vi "Test Drive.vi"   [LabVIEW 2016]
uses:
  <vilib>/Rock Robotics/WPI/ThirdParty/CanMotor/TalonSRX/WPI_CANTalonSRX_APIControlMode.ctl
  <vilib>/Rock Robotics/WPI/Solenoid/WPI_SolenoidValue.ctl
  Global Variables/Refnum Names.vi
  <vilib>/Rock Robotics/WPI/Utilities/WPI_GetSetVariantRefNum.vi
  <vilib>/Rock Robotics/WPI/Joystick/WPI_JoystickArcadeMapping.vi
  <vilib>/Rock Robotics/WPI/Solenoid/WPI_SolenoidSetEnum.vi
types:
  T1 = typedef "WPI_CANTalonSRX_APIControlMode.ctl" = enum8{"Percent VBus", "Speed", "Position", "Slave", "Unchanged / Invalid", "Voltage Compensation", "Current", "Motion Profile", "Motion Magic"}
  T2 = typedef "WPI_MotorControlDeviceRef.ctl" = cluster{"DeviceStatus":errorcluster, "Type":T3, "PWM":cluster{"PWM Channel":T4, "DeadBand":T5}, "CAN":cluster{"Device Number":u8, "SetOutput VI Ref":variant, "GetOutput VI Ref":variant, "Enable VI Ref":variant, "Disable VI Ref":variant, "Data":variant}, "Invert":bool}
  T3 = typedef "WPI_MotorControlType.ctl" = enum16{"PWM", "CAN"}
  T4 = typedef "FPGA_DIOPWMChannel.ctl" = enum8{"PWM 0", "PWM 1", "PWM 2", "PWM 3", "PWM 4", "PWM 5", "PWM 6", "PWM 7", "PWM 8", "PWM 9", "PWM MXP 0", "PWM MXP 1", "PWM MXP 2", "PWM MXP 3", "PWM MXP 4", "PWM MXP 5", "PWM MXP 6", "PWM MXP 7", "PWM MXP 8", "PWM MXP 9", "Invalid"}
  T5 = typedef "WPI_PWMDeadband.ctl" = cluster{"Name":string, "maxPositivePwm":i32, "minPositivePwm":i32, "centerPwm":i32, "maxNegativePwm":i32, "minNegativePwm":i32, "angularRange":u16}
  T6 = typedef "WPI_JoystickDevRef.ctl" = cluster{"Device":T7}
  T7 = typedef "WPI_JoystickDeviceEnum.ctl" = enum16{"USB 0", "USB 1", "USB 2", "USB 3", "USB 4", "USB 5"}
  T8 = typedef "WPI_SolenoidDevRef.ctl" = cluster{"DevStatus":errorcluster, "Pneumatics Control Module":u8, "Forward Solenoid Channel":T9, "Reverse Solenoid Channel":T9}
  T9 = typedef "WPI_SolenoidChannel.ctl" = enum8{"Solenoid 0", "Solenoid 1", "Solenoid 2", "Solenoid 3", "Solenoid 4", "Solenoid 5", "Solenoid 6", "Solenoid 7", "Invalid"}
  T10 = typedef "WPI_SolenoidValue.ctl" = enum16{"Off", "On", "Forward", "Reverse"}
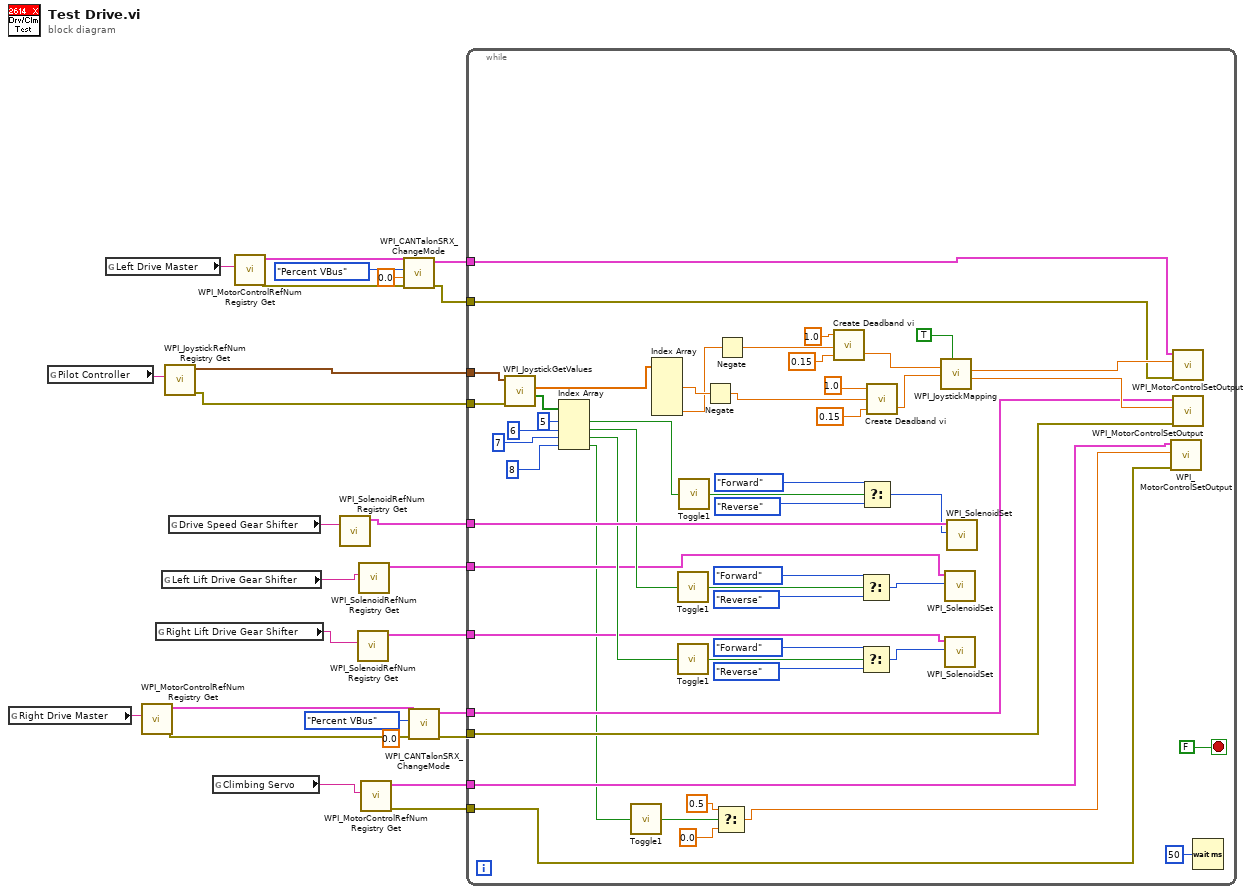
[diagram p0: block diagram]
diagram:
  n1 = global read "Refnum Names.vi" "Right Drive Master"() -> (w25:string)
  n2 = global read "Refnum Names.vi" "Pilot Controller"() -> (w24:string)
  n3 = global read "Refnum Names.vi" "Left Drive Master"() -> (w26:string)
  n4 = call <vilib>:"WPI_MotorControlRefNum Registry Get.vi"("refnum name"=w25) -> ("error out"=w17:errorcluster, "MotorControlDevRef"=w18:T2)  [unwired: 9 in]
  n5 = global read "Refnum Names.vi" "Right Lift Drive Gear Shifter"() -> (w8:string)
  n6 = global read "Refnum Names.vi" "Left Lift Drive Gear Shifter"() -> (w9:string)
  n7 = call <vilib>:"WPI_JoystickRefNum Registry Get.vi"("refnum name"=w24) -> ("error out"=w12:errorcluster, "JoystickDevRef"=w13:T6)  [unwired: 9 in]
  n8 = global read "Refnum Names.vi" "Drive Speed Gear Shifter"() -> (w11:string)
  n9 = global read "Refnum Names.vi" "Climbing Servo"() -> (w5:string)
  n10 = call <vilib>:"WPI_MotorControlRefNum Registry Get.vi"("refnum name"=w26) -> ("error out"=w22:errorcluster, "MotorControlDevRef"=w23:T2)  [unwired: 9 in]
  n11 = call <vilib>:"WPI_SolenoidRefNum Registry Get.vi"("refnum name"=w11) -> ("SolenoidDevRef"=w10:T8)  [unwired: 9 in, 1 out]
  n12 = call <vilib>:"WPI_SolenoidRefNum Registry Get.vi"("refnum name"=w8) -> ("SolenoidDevRef"=w6:T8)  [unwired: 9 in, 1 out]
  n13 = call <vilib>:"WPI_SolenoidRefNum Registry Get.vi"("refnum name"=w9) -> ("SolenoidDevRef"=w7:T8)  [unwired: 9 in, 1 out]
  n14 = call <vilib>:"WPI_MotorControlRefNum Registry Get.vi"("refnum name"=w5) -> ("error out"=w3:errorcluster, "MotorControlDevRef"=w4:T2)  [unwired: 9 in]
  n15 = call <vilib>:"WPI_CANTalonSRX_ChangeMode.vi"("error in (no error)"=w22, "Output"=0.0, "Control Mode"=WPI_CANTalonSRX_APIControlMode."Percent VBus", "CAN Talon SRX Ref"=w23) -> ("error out"=w19:errorcluster, "CAN Talon SRX Ref"=w20:T2)  [unwired: 6 in]
  n16 = call <vilib>:"WPI_CANTalonSRX_ChangeMode.vi"("error in (no error)"=w17, "Output"=0.0, "Control Mode"=WPI_CANTalonSRX_APIControlMode."Percent VBus", "CAN Talon SRX Ref"=w18) -> ("error out"=w15:errorcluster, "CAN Talon SRX Ref"=w16:T2)  [unwired: 6 in]
  n17 = while {
    tunnel: w20 -> [w75]
    tunnel: w19 -> [w74]
    tunnel: w16 -> [w73]
    tunnel: w15 -> [w72]
    tunnel: w13 -> [w59]
    tunnel: w12 -> [w58]
    tunnel: w10 -> [w56]
    tunnel: w7 -> [w36]
    tunnel: w6 -> [w35]
    tunnel: w4 -> [w33]
    tunnel: w3 -> [w27]
    stop <- FALSE stop-if-true
    n18 = call <vilib>:"WPI_JoystickGetValues.vi"("error in (no error)"=w58, "JoystickDevRef"=w59) -> ("Buttons"=w55:bool[], "Axes"=w60:dbl[])  [unwired: 5 in, 3 out]
    n19 = Index Array(array=w55, index #1=5 ("index"), index #2=6 ("index"), index #3=7 ("index"), index #4=8 ("index")) -> (element #1=w54:bool, element #2=w43:bool, element #3=w39:bool, element #4=w32:bool)
    n20 = call "Toggle1.vi"("Boolean"=w32) -> ("Driver Switch 2"=w31:bool)
    n21 = Index Array(array=w60) -> (element #2=w76:dbl, element #5=w71:dbl)  [unwired: 5 in, 3 out]
    n22 = call "Toggle1.vi"("Boolean"=w43) -> ("Driver Switch 2"=w44:bool)
    n23 = call "Toggle1.vi"("Boolean"=w39) -> ("Driver Switch 2"=w42:bool)
    n24 = call "Toggle1.vi"("Boolean"=w54) -> ("Driver Switch 2"=w53:bool)
    n25 = Negate(x=w76) -> (-x=w70:dbl)
    n26 = Select(t=0.5, s=w31, f=0.0) -> (s? t:f=w28:dbl)
    n27 = Negate(x=w71) -> (-x=w57:dbl)
    n28 = call "Create Deadband vi.vi"("Input Deadband"=0.15 ("Output Upper Limit"), "Input"=w57, "Output Upper Limit"=1.0) -> ("Output"=w68:dbl)  [unwired: 1 in]
    n29 = Select(t=WPI_SolenoidValue."Forward" ("Value"), s=w44, f=WPI_SolenoidValue."Reverse" ("Value")) -> (s? t:f=w37:T10)
    n30 = Select(t=WPI_SolenoidValue."Forward" ("Value"), s=w42, f=WPI_SolenoidValue."Reverse" ("Value")) -> (s? t:f=w38:T10)
    n31 = Select(t=WPI_SolenoidValue."Forward" ("Value"), s=w53, f=WPI_SolenoidValue."Reverse" ("Value")) -> (s? t:f=w51:T10)
    n32 = call "Create Deadband vi.vi"("Input Deadband"=0.15 ("Output Upper Limit"), "Input"=w70, "Output Upper Limit"=1.0) -> ("Output"=w69:dbl)  [unwired: 1 in]
    n33 = call-poly <vilib>:"WPI_JoystickMapping.vi"("Square Inputs"=TRUE, "Y axis value"=w69, "X axis value"=w68) -> ("Right Motor Value"=w77:dbl, "Left Motor Value"=w78:dbl)  [unwired: 7 in]
    n34 = call-poly <vilib>:"WPI_SolenoidSet.vi"("Value"=w37, "SolenoidDevRef"=w36) -> ()  [unwired: 8 in, 2 out]
    n35 = call-poly <vilib>:"WPI_SolenoidSet.vi"("Value"=w38, "SolenoidDevRef"=w35) -> ()  [unwired: 8 in, 2 out]
    n36 = call-poly <vilib>:"WPI_SolenoidSet.vi"("Value"=w51, "SolenoidDevRef"=w56) -> ()  [unwired: 8 in, 2 out]
    n37 = call <vilib>:"WPI_MotorControlSetOutput.vi"("error in (no error)"=w27, "Output"=w28, "MotorControlDevRef"=w33) -> ()  [unwired: 6 in, 3 out]
    n38 = call <vilib>:"WPI_MotorControlSetOutput.vi"("error in (no error)"=w74, "Output"=w78, "MotorControlDevRef"=w75) -> ()  [unwired: 6 in, 3 out]
    n39 = call <vilib>:"WPI_MotorControlSetOutput.vi"("error in (no error)"=w72, "Output"=w77, "MotorControlDevRef"=w73) -> ()  [unwired: 6 in, 3 out]
    n40 = Wait (ms)(milliseconds to wait=u32 50) -> ()  [unwired: 1 out]
  }
